vi "CODMn固定站质控流程 (子VI).vi"(9 "CODMn量程切换":enum32{"H", "L", "AUTO"}(ring)=enum."AUTO", 10 "CODMn":bool) -> (2 "CODMn中断报警":bool, 3 "布尔":bool)   [LabVIEW 2016, in "质控单元.lvlib"]
panel:
  out "参数 out":T1
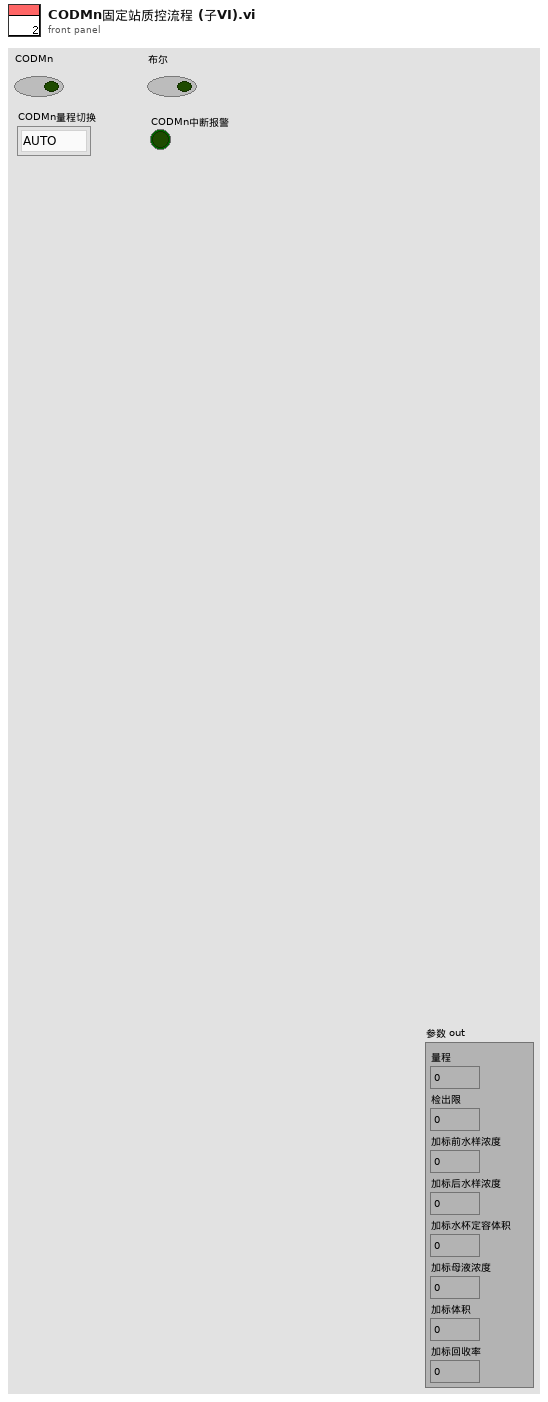
[diagram p1: front panel]
types:
  T1 = cluster{"量程":dbl, "检出限":dbl, "加标前水样浓度":dbl, "加标后水样浓度":dbl, "加标水杯定容体积":dbl, "加标母液浓度":dbl, "加标体积":dbl, "加标回收率":dbl}
  T2 = enum16{"待机", "启动水样测量", "水样测量中", "启动加标", "启动加标回收", "加标回收测量中", "结束"}
  T3 = cluster{"测量模式":enum16{"水样测量", "标样核查", "零点核查", "跨度核查", "空白测试", "加标回收", "平行样", "校零", "校标"}}
  T4 = enum16{"空闲", "水样测试", "标样核查", "零点核查", "跨度核查", "空白测试", "平行样测试", "质控样", "空白校准", "标样校准", "加标回收"}
  T5 = enum16{"空闲", "水样测试", "标样核查", "零点核查", "跨度核查", "空白测试", "平行样测试", "加标回收", "空白校准", "标样校准", "初始化（清洗）"}
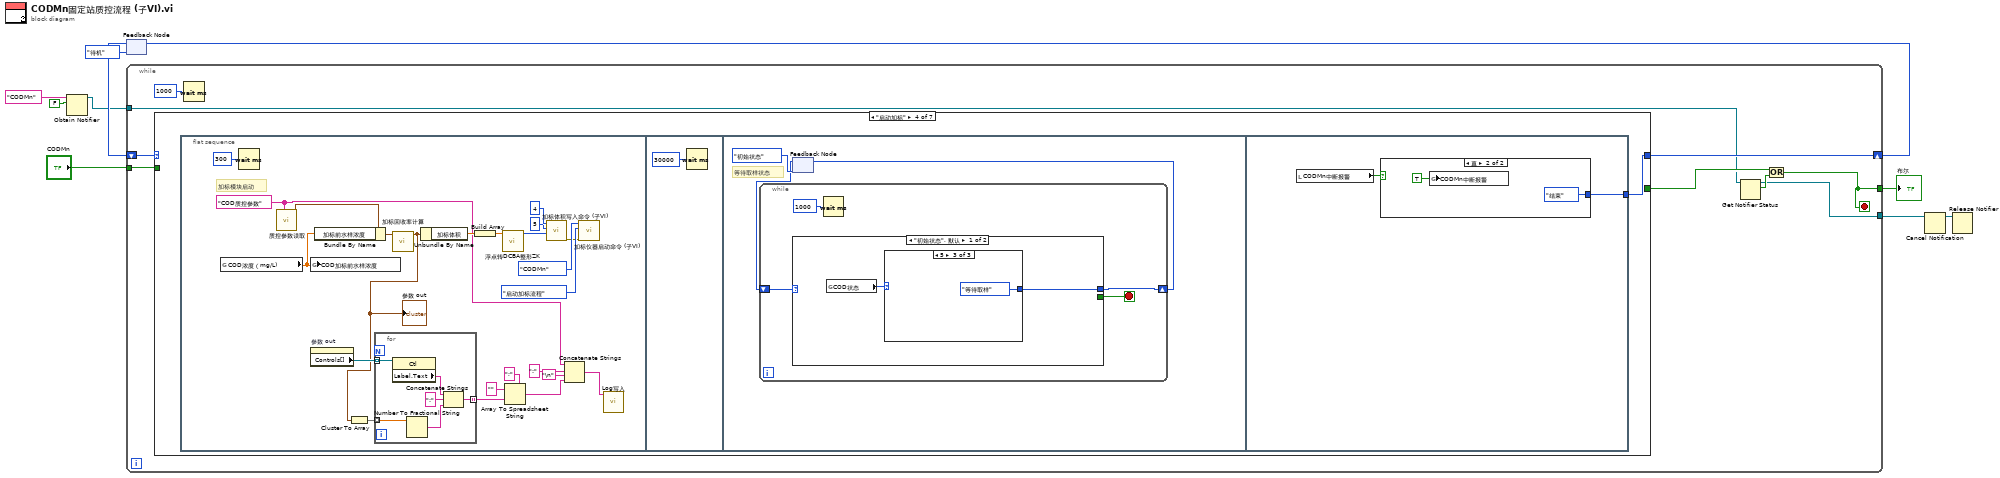
[diagram p0: block diagram]
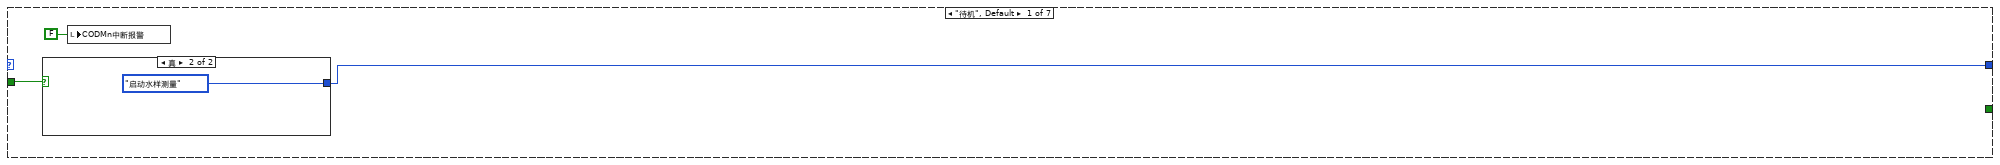
[diagram p2: hidden frame]
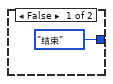
[diagram p3: hidden frame]
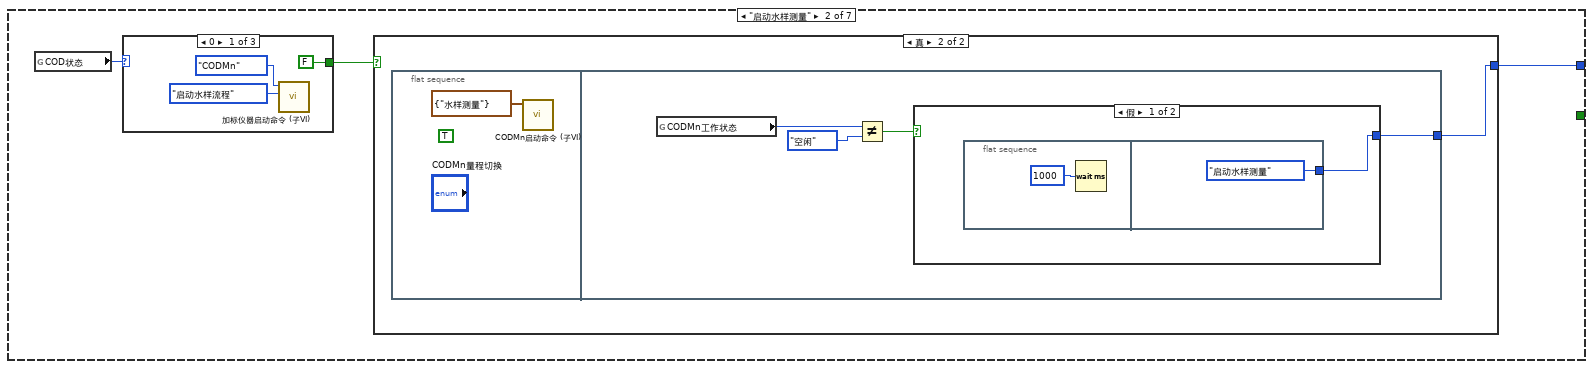
[diagram p4: hidden frame]
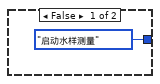
[diagram p5: hidden frame]
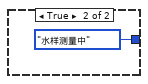
[diagram p6: hidden frame]
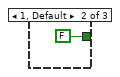
[diagram p7: hidden frame]
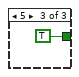
[diagram p8: hidden frame]
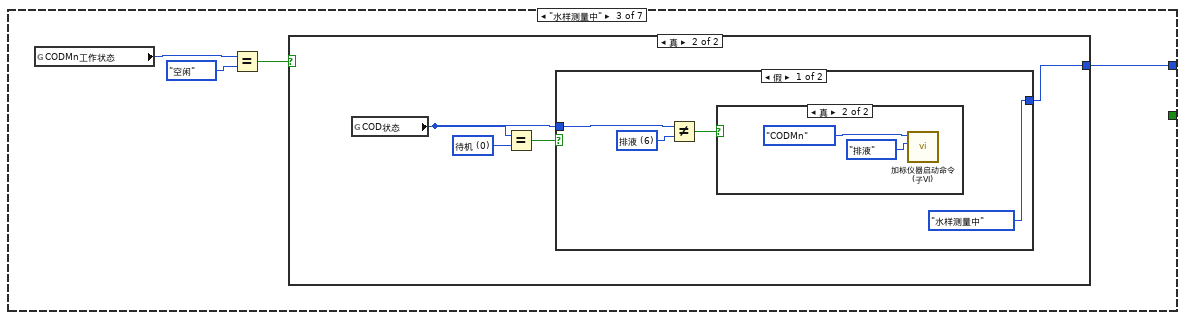
[diagram p9: hidden frame]
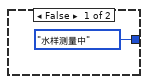
[diagram p10: hidden frame]
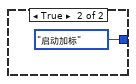
[diagram p12: hidden frame]
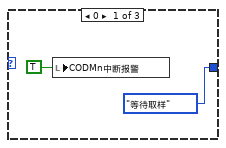
[diagram p13: hidden frame]
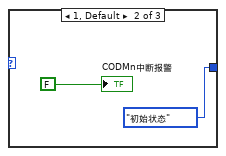
[diagram p14: hidden frame]
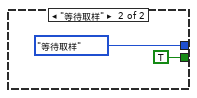
[diagram p15: hidden frame]
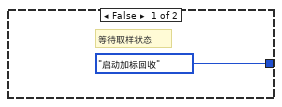
[diagram p16: hidden frame]
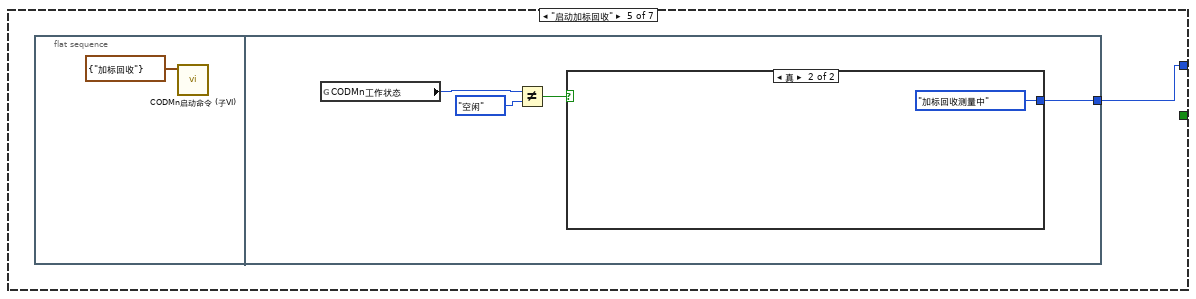
[diagram p17: hidden frame]
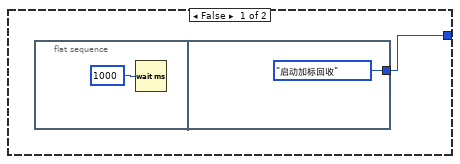
[diagram p18: hidden frame]
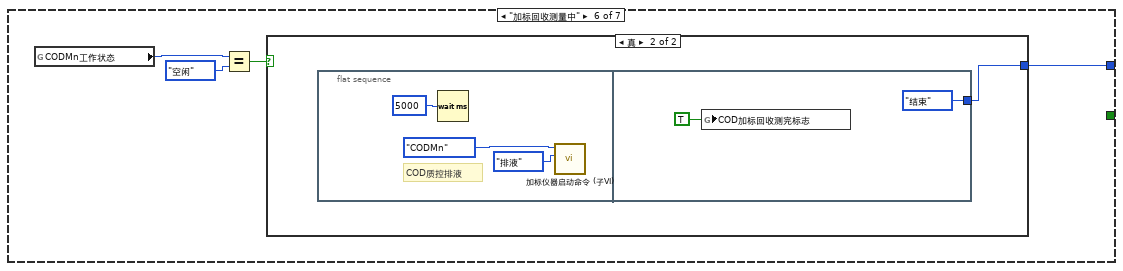
[diagram p19: hidden frame]
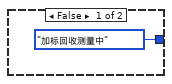
[diagram p20: hidden frame]
diagram:
  n1 = Obtain Notifier(name (unnamed)="CODMn" ("名称（未命名）"), notification data type=FALSE) -> (notifier out=w3:refnum<notifier>)  [unwired: 2 in, 2 out]
  n2 = feedback #1(T2."待机") -> (w6:T2)
  n3 = while {
    tunnel: "CODMn" -> [w19]
    tunnel: [w13] -> w8
    shift-right: [w18] -> w9
    shift-left: w6 -> [w17]
    tunnel: w3 -> [w12]
    tunnel: [w11] -> w1
    stop <- w13 stop-if-true
    n4 = case shown="\"启动加标\"" w17 {
      tunnel: [w22 w27 w47 w60 w112 w125 T2."结束"] -> w18
      tunnel: [_ _ _ _ _ _ TRUE] -> w14
      tunnel: w19 -> [w21 _ _ _ _ _ _]
      frame "待机", Default {
        n5 = case shown="真" w21 {
          tunnel: [T2."结束" T2."启动水样测量"] -> w22
          frame False {
          }
          frame True {
          }
        }
        n6 = local write "CODMn中断报警"(FALSE ("CODMn中断报警")) -> ()
      }
      frame "启动水样测量" {
        n7 = global read "加标回收状态全局变量.vi" "COD状态"() -> (w26:u16)
        n8 = case shown="0" w26 {
          tunnel: [FALSE ("s") FALSE ("s") TRUE ("s")] -> w25
          frame 0 {
            n9 = call "加标仪器启动命令 (子VI).vi"("启动命令"=enum16{"启动水样流程", "启动加标流程", "排液", "停止"}."启动水样流程", "仪器"=enum16{"", "氨氮", "总磷", "总氮", "CODMn", "CODCr"}."CODMn") -> ()  [unwired: 9 in, 1 out]
          }
          frame 1, Default {
          }
          frame 5 {
          }
        }
        n10 = case shown="真" w25 {
          tunnel: [T2."启动水样测量" w29] -> w27
          frame False {
          }
          frame True {
            n11 = flat-sequence {
              tunnel: [w34] -> w29
              frame #0 {
                (unwired) TRUE ("强制切换")
                n12 = call "CODMn启动命令 (子VI).vi"("启动测量模式"=T3 {"测量模式"=enum."水样测量"}) -> ()  [unwired: 10 in, 1 out]
              }
              frame #1 {
                n13 = global read "与CODMn交互全局.vi" "CODMn工作状态"() -> (w33:T5)
                n14 = Not Equal?(x=w33, y=T4."空闲") -> (x != y?=w31:bool)
                n15 = case shown="假" w31 {
                  tunnel: [w35 T2."水样测量中"] -> w34
                  frame False {
                    n16 = flat-sequence {
                      tunnel: [T2."启动水样测量"] -> w35
                      frame #0 {
                        n17 = Wait (ms)(milliseconds to wait=u32 1000 ("等待时间（毫秒）")) -> ()  [unwired: 1 out]
                      }
                      frame #1 {
                      }
                    }
                  }
                  frame True {
                  }
                }
              }
            }
          }
        }
      }
      frame "水样测量中" {
        n18 = global read "与CODMn交互全局.vi" "CODMn工作状态"() -> (w46:T5)
        n19 = Equal?(x=w46, y=T4."空闲") -> (x = y?=w44:bool)
        n20 = case shown="真" w44 {
          tunnel: [T2."水样测量中" w52] -> w47
          frame False {
          }
          frame True {
            w51 = u16 0 items=["待机", "润洗", "进样", "进样完成", "柱塞泵加标", "等待取液", "排液"] ("COD状态")
            n21 = global read "加标回收状态全局变量.vi" "COD状态"() -> (w49:u16)
            n22 = Equal?(x=w49, y=w51) -> (x = y?=w50:bool)
            n23 = case shown="假" w50 {
              tunnel: [T2."水样测量中" T2."启动加标"] -> w52
              tunnel: w49 -> [w54 _]
              frame False {
                w55 = u16 6 items=["待机", "润洗", "进样", "进样完成", "柱塞泵加标", "等待取液", "排液"] ("氨氮状态")
                n24 = Not Equal?(x=w54, y=w55) -> (x != y?=w53:bool)
                n25 = case shown="真" w53 {
                  frame False {
                  }
                  frame True {
                    n26 = call "加标仪器启动命令 (子VI).vi"("启动命令"=enum16{"启动水样流程", "启动加标流程", "排液", "停止"}."排液", "仪器"=enum16{"", "氨氮", "总磷", "总氮", "CODMn", "CODCr"}."CODMn") -> ()  [unwired: 9 in, 1 out]
                  }
                }
              }
              frame True {
              }
            }
          }
        }
      }
      frame "启动加标" {
        n27 = flat-sequence {
          tunnel: [w108] -> w60
          frame #0 {
            w62 = "COD质控参数" ("section")
            # "加标模块启动"
            n28 = global read "与CODMn交互全局.vi" "COD浓度（mg/L)"() -> (w80:dbl)
            n29 = Wait (ms)(milliseconds to wait=u32 300 ("等待时间（毫秒）")) -> ()  [unwired: 1 out]
            n30 = call "质控参数读取.vi"("section"=w62) -> ("参数"=w82:T1)  [unwired: 9 in, 1 out]
            n31 = global write "水样浓度全局.vi" "COD加标前水样浓度"(w80) -> ()
            n32 = property on="参数 out" class="Clust (严格)"() -> ("Controls[]"=w67:refnum<vi>[])  [unwired: 2 in, 2 out]
            n33 = Bundle By Name(cluster=w82, "加标前水样浓度"=w80) -> (w83:T1)
            n34 = call "加标回收率计算.vi"("参数"=w83) -> ("参数 out"=w61:T1)  [unwired: 9 in, 1 out]
            "参数 out" <- w61
            n35 = Cluster To Array(cluster=w61) -> (array=w69:dbl[])
            n36 = for {
              tunnel: w67 -> [w89] mode=indexing
              tunnel: w69 -> [w87] mode=indexing
              tunnel: [w84] -> w68 mode=indexing
              n37 = property class="Ctl"(reference=w89) -> ("Label.Text"=w88:string)  [unwired: 1 in, 2 out]
              n38 = Number To Fractional String(number=w87) -> (F-format string=w85:string)  [unwired: 3 in]
              n39 = Concatenate Strings(w88, ":" ("字符串"), w85) -> (w84:string)
            }
            n40 = Unbundle By Name(w61) -> ("加标体积"=w81:dbl)
            n41 = Build Array(w81) -> (w78:dbl[])
            n42 = call "浮点转DCBA整形ZK.vi"("浮点数"=w78) -> ("DCBA整形输出"=w73:u16[])  [unwired: 10 in]
            n43 = Array To Spreadsheet String(delimiter (Tab)=";" ("分隔符(Tab)"), array=w68, 3:"") -> (spreadsheet string=w65:string)
            n44 = call "加标体积写入命令 (子VI).vi"("values"=w73, "starting address"=u16 5, "Slave ID"=u16 4 ("value")) -> ("错误输出"=w72:errorcluster)  [unwired: 8 in]
            n45 = Concatenate Strings(w62, ":" ("字符串"), "\n", w65) -> (w63:string)
            n46 = call "加标仪器启动命令 (子VI).vi"("错误输入（无错误）"=w72, "启动命令"=enum16{"启动水样流程", "启动加标流程", "排液", "停止"}."启动加标流程", "仪器"=enum16{"", "氨氮", "总磷", "总氮", "CODMn", "CODCr"}."CODMn") -> ()  [unwired: 8 in, 1 out]
            n47 = call "Log写入.vi"("Log"=w63) -> ()  [unwired: 11 in]
          }
          frame #1 {
            n48 = Wait (ms)(milliseconds to wait=u32 30000 ("等待时间（毫秒）")) -> ()  [unwired: 1 out]
          }
          frame #2 {
            # "等待取样状态"
            n49 = feedback #2(enum16{"初始状态", "等待取样"}."初始状态") -> (w92:enum16{"初始状态", "等待取样"})
            n50 = while {
              shift-right: [w96] -> w91
              shift-left: w92 -> [w97]
              stop <- w95 stop-if-true
              n51 = case shown="\"初始状态\", 默认" w97 {
                tunnel: [w99 enum16{"初始状态", "等待取样"}."等待取样"] -> w96
                tunnel: [_ TRUE] -> w95
                frame "初始状态", Default {
                  n52 = global read "加标回收状态全局变量.vi" "COD状态"() -> (w98:u16)
                  n53 = case shown="5" w98 {
                    tunnel: [enum16{"初始状态", "等待取样"}."等待取样" enum16{"初始状态", "等待取样"}."初始状态" enum16{"初始状态", "等待取样"}."等待取样"] -> w99
                    frame 0 {
                      n54 = local write "CODMn中断报警"(TRUE ("氨氮中断报警")) -> ()
                    }
                    frame 1, Default {
                      "CODMn中断报警" <- FALSE ("总氮中断报警")
                    }
                    frame 5 {
                    }
                  }
                }
                frame "等待取样" {
                }
              }
              n55 = Wait (ms)(milliseconds to wait=u32 1000 ("等待时间（毫秒）")) -> ()  [unwired: 1 out]
            }
            n56 = feedback-in #2(w91) -> ()
          }
          frame #3 {
            n57 = local read "CODMn中断报警"() -> (w107:bool)
            n58 = case shown="真" w107 {
              tunnel: [T2."启动加标回收" T2."结束"] -> w108
              frame False {
                # "等待取样状态"
              }
              frame True {
                n59 = global write "质控中断报警全局.vi" "CODMn中断报警"(TRUE ("CODMn中断报警")) -> ()
              }
            }
          }
        }
      }
      frame "启动加标回收" {
        n60 = flat-sequence {
          tunnel: [w117] -> w112
          frame #0 {
            n61 = call "CODMn启动命令 (子VI).vi"("启动测量模式"=T3 {"测量模式"=enum."加标回收"}) -> ()  [unwired: 10 in, 1 out]
          }
          frame #1 {
            n62 = global read "与CODMn交互全局.vi" "CODMn工作状态"() -> (w116:T5)
            n63 = Not Equal?(x=w116, y=T4."空闲") -> (x != y?=w114:bool)
            n64 = case shown="真" w114 {
              tunnel: [w118 T2."加标回收测量中"] -> w117
              frame False {
                n65 = flat-sequence {
                  tunnel: [T2."启动加标回收"] -> w118
                  frame #0 {
                    n66 = Wait (ms)(milliseconds to wait=u32 1000 ("等待时间（毫秒）")) -> ()  [unwired: 1 out]
                  }
                  frame #1 {
                  }
                }
              }
              frame True {
              }
            }
          }
        }
      }
      frame "加标回收测量中" {
        n67 = global read "与CODMn交互全局.vi" "CODMn工作状态"() -> (w124:T5)
        n68 = Equal?(x=w124, y=T4."空闲") -> (x = y?=w122:bool)
        n69 = case shown="真" w122 {
          tunnel: [T2."加标回收测量中" w127] -> w125
          frame False {
          }
          frame True {
            n70 = flat-sequence {
              tunnel: [T2."结束"] -> w127
              frame #0 {
                # "COD质控排液"
                n71 = Wait (ms)(milliseconds to wait=u32 5000 ("等待时间（毫秒）")) -> ()  [unwired: 1 out]
                n72 = call "加标仪器启动命令 (子VI).vi"("启动命令"=enum16{"启动水样流程", "启动加标流程", "排液", "停止"}."排液", "仪器"=enum16{"", "氨氮", "总磷", "总氮", "CODMn", "CODCr"}."CODMn") -> ()  [unwired: 9 in, 1 out]
              }
              frame #1 {
                n73 = global write "质控测完标志全局 1.vi" "COD加标回收测完标志"(TRUE ("COD加标回收测完标志")) -> ()
              }
            }
          }
        }
      }
      frame "结束" {
        n74 = Wait (ms)(milliseconds to wait=u32 5000 ("等待时间（毫秒）")) -> ()  [unwired: 1 out]
      }
    }
    n75 = Wait (ms)(milliseconds to wait=u32 1000 ("等待时间（毫秒）")) -> ()  [unwired: 1 out]
    n76 = Get Notifier Status(notifier=w12) -> (notifier out=w11:refnum<notifier>, current notification=w15:bool)  [unwired: 1 in, 3 out]
    n77 = Or(x=w14, y=w15) -> (x .or. y?=w13:bool)
  }
  "布尔" <- w8
  n78 = feedback-in #1(w9) -> ()
  n79 = Cancel Notification(0:w1) -> (8:w2:refnum<notifier>)  [unwired: 1 in, 2 out]
  n80 = Release Notifier(notifier=w2) -> ()  [unwired: 2 in, 3 out]
